vi "Exercise4.1-Pre-Lab1.vi"() -> ()   [LabVIEW 2013]
uses:
  <vilib>/measure/NI_MABase.lvlib
panel:
  in  "Enum":T1(ring)
  in  "stop":bool
  out "Waveform Graph":waveform(dbl)(graph)={"t0"=timestamp(0 s since 1904-01-01), "dt"=0.00025, "Y"=[0.0, 0.15643446504023087, 0.30901699437494745, 0.4539904997395468, 0.5877852522924731, 0.7071067811865476, 0.8090169943749475, 0.8910065241883679, 0.9510565162951536, 0.9876883405951378, 1.0, 0.9876883405951378, 0.9510565162951535, 0.8910065241883679, 0.8090169943749473, 0.7071067811865476, 0.587785252292473, 0.4539904997395468, 0.30901699437494734, 0.15643446504023084, -5.21772295508649e-17, -0.15643446504023092, -0.30901699437494745, -0.45399049973954686, -0.5877852522924731, -0.7071067811865476, -0.8090169943749473, -0.8910065241883679, -0.9510565162951534, -0.9876883405951378, -0.9999999999999998, -0.9876883405951378, -0.9510565162951533, -0.8910065241883679, -0.8090169943749472, -0.7071067811865476, -0.587785252292473, -0.4539904997395468, -0.3090169943749474, -0.15643446504023087, -3.4314998759166215e-17, 0.15643446504023087, 0.30901699437494734, 0.4539904997395468, 0.587785252292473, 0.7071067811865476, 0.8090169943749472, 0.8910065241883679, 0.9510565162951533, 0.9876883405951378, 0.9999999999999998, 0.9876883405951378, 0.9510565162951534, 0.8910065241883679, 0.8090169943749473, 0.7071067811865476, 0.5877852522924731, 0.4539904997395468, 0.3090169943749475, 0.15643446504023087, 1.2284010614260765e-16, -0.1564344650402309, -0.3090169943749473, -0.4539904997395468, -0.587785252292473, -0.7071067811865476, -0.8090169943749473, -0.8910065241883679, -0.9510565162951535, -0.9876883405951378, -1.0, -0.9876883405951378, -0.9510565162951535, -0.8910065241883679, -0.8090169943749473, -0.7071067811865476, -0.587785252292473, -0.4539904997395468, -0.30901699437494734, -0.15643446504023087, 4.512991542970912e-17, 0.1564344650402309, 0.30901699437494745, 0.45399049973954686, 0.5877852522924731, 0.7071067811865476, 0.8090169943749473, 0.8910065241883679, 0.9510565162951534, 0.9876883405951378, 0.9999999999999998, 0.9876883405951378, 0.9510565162951533, 0.8910065241883679, 0.8090169943749472, 0.7071067811865476, 0.587785252292473, 0.4539904997395468, 0.3090169943749474, 0.15643446504023087]}
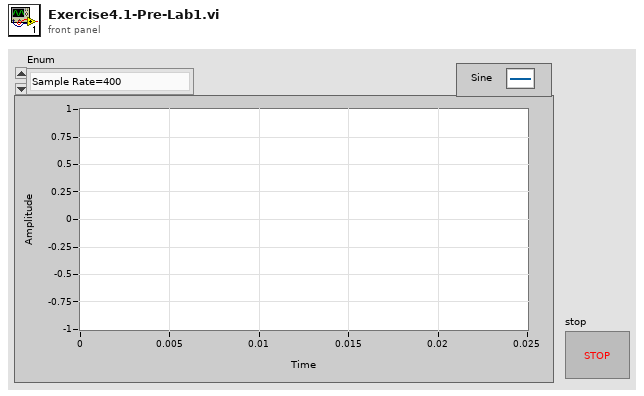
[diagram p1: front panel]
types:
  T1 = enum16{"Sample Rate=400", "Sample Rate=1000", "Sample Rate=4000"}
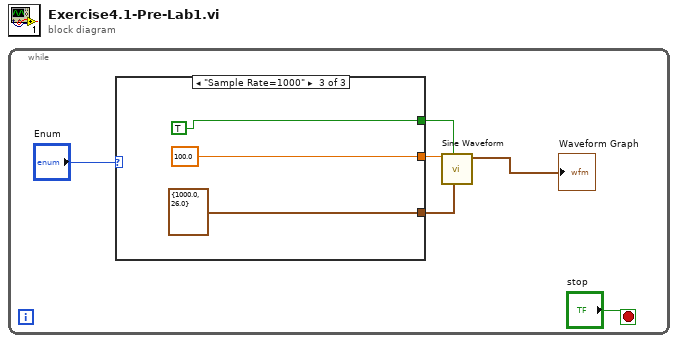
[diagram p0: block diagram]
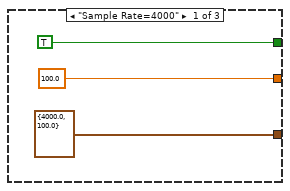
[diagram p2: hidden frame]
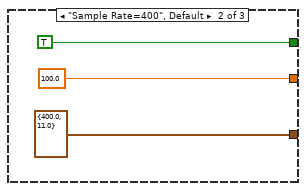
[diagram p3: hidden frame]
diagram:
  n1 = while {
    stop <- "stop" stop-if-true
    n2 = case shown="\"Sample Rate=1000\"" "Enum" {
      tunnel: [TRUE ("reset signal") TRUE ("reset signal") TRUE ("reset signal")] -> w1
      tunnel: [100.0 ("frequency") 100.0 ("frequency") 100.0 ("frequency")] -> w3
      tunnel: [cluster{"Fs":dbl, "#s":dbl} {"Fs"=4000.0, "#s"=100.0} ("sampling info") cluster{"Fs":dbl, "#s":dbl} {"Fs"=400.0, "#s"=11.0} ("sampling info") cluster{"Fs":dbl, "#s":dbl} {"Fs"=1000.0, "#s"=26.0} ("sampling info")] -> w2
      frame "Sample Rate=4000" {
      }
      frame "Sample Rate=400", Default {
      }
      frame "Sample Rate=1000" {
      }
    }
    n3 = call <vilib>:"Sine Waveform.vi"("sampling info"=w2, "reset signal"=w1, "frequency"=w3) -> ("signal out"=→"Waveform Graph":waveform(dbl))  [unwired: 7 in, 1 out]
  }
